vi "Create Listen Events.vi"(8 "error in (no error)":errorcluster, 11 "CIFCorePlugin in":refnum<class "CIFCorePlugin.lvclass">) -> (0 "error out":errorcluster, 3 "CIFCorePlugin out":refnum<class "CIFCorePlugin.lvclass">)   [LabVIEW 2021, in "CIFCorePlugin.lvclass"]
uses:
  CIFCorePlugin.lvclass
  CIFCorePlugin.lvclass/CIFCorePlugin.ctl
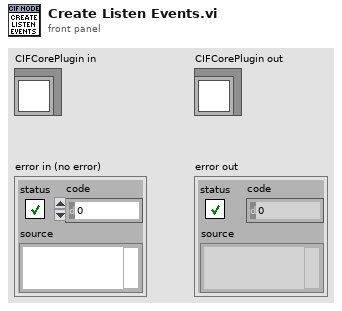
[diagram p1: front panel]
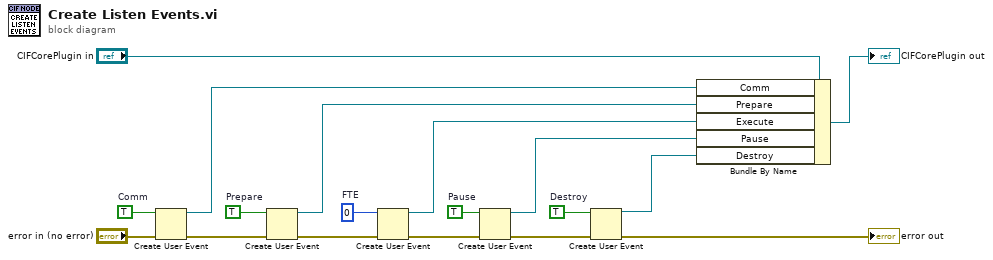
[diagram p0: block diagram]
diagram:
  w1 = i64 0  # FTE
  w13 = TRUE  # Destroy
  w14 = TRUE  # Pause
  w15 = TRUE  # Prepare
  w16 = TRUE  # Comm
  n1 = Create User Event(user event datatype=w16, error in="error in (no error)") -> (user event=w2:refnum<user-event>, error out=w12:errorcluster)
  n2 = Create User Event(user event datatype=w15, error in=w12) -> (user event=w3:refnum<user-event>, error out=w11:errorcluster)
  n3 = Create User Event(user event datatype=w1, error in=w11) -> (user event=w4:refnum<user-event>, error out=w10:errorcluster)
  n4 = Create User Event(user event datatype=w14, error in=w10) -> (user event=w5:refnum<user-event>, error out=w9:errorcluster)
  n5 = Create User Event(user event datatype=w13, error in=w9) -> (user event=w6:refnum<user-event>, error out=→"error out":errorcluster)
  n6 = Bundle By Name(cluster="CIFCorePlugin in", "Comm"=w2, "Prepare"=w3, "Execute"=w4, "Pause"=w5, "Destroy"=w6) -> (→"CIFCorePlugin out":refnum<class "CIFCorePlugin.lvclass">)
